vi "IsRequired.vi"(8 "error in":errorcluster, 11 "Control Terminal in":refnum<class "ControlTerminal.lvclass">) -> (0 "error out":errorcluster, 2 "required":bool, 3 "Control Terminal out":refnum<class "ControlTerminal.lvclass">)   [LabVIEW 2014, in "ControlTerminal.lvclass"]
uses:
  ControlTerminal.lvclass
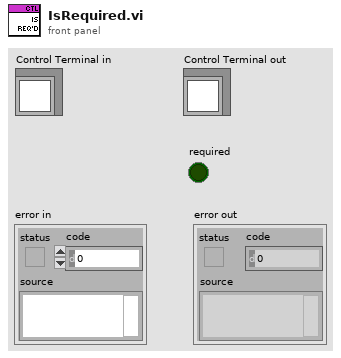
[diagram p1: front panel]
types:
  T1 = enum16{"Invalid Wire Rule", "Required", "Recommended", "Optional", "Dynamic Dispatch"}
  T2 = enum16{"Invalid Wire Rule", "Required", "Recommended", "Optional", "Dynamic Dispatch"}[]
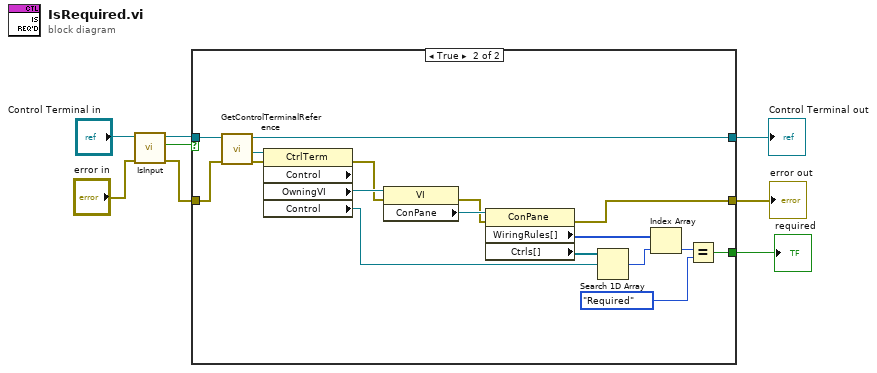
[diagram p0: block diagram]
diagram:
  n1 = call-dynamic "IsInput.vi"("error in"="error in", "ControlTerminal in"="Control Terminal in") -> ("error out"=w2:errorcluster, "input"=w3:bool, "ControlTerminal out"=w4:refnum<class "ControlTerminal.lvclass">)  [unwired: 5 in]
  n2 = case shown="True" w3 {
    tunnel: [w9 w16] -> w8
    tunnel: [_ w17] -> w7
    tunnel: w4 -> [w10 w15]
    tunnel: w2 -> [w9 w14]
    tunnel: [w10 w11] -> w6
    frame False {
    }
    frame True {
      n3 = call "GetControlTerminalReference.vi"("error in"=w14, "ControlTerminal in"=w15) -> ("error out"=w13:errorcluster, "reference"=w12:refnum<vi>, "ControlTerminal out"=w11:refnum<class "ControlTerminal.lvclass">)  [unwired: 7 in]
      n4 = property class="CtrlTerm" props=["Control", "OwningVI", "Control"](reference=w12, error in=w13) -> (error out=w24:errorcluster, "OwningVI"=w27:refnum<vi>, "Control"=w22:refnum<vi>)  [unwired: 2 out]
      n5 = property class="VI"(reference=w27, error in=w24) -> (error out=w25:errorcluster, "ConPane"=w26:refnum<vi>)  [unwired: 1 out]
      n6 = property class="ConPane"(reference=w26, error in=w25) -> (error out=w16:errorcluster, "WiringRules[]"=w21:T2, "Ctrls[]"=w23:refnum<vi>[])  [unwired: 1 out]
      n7 = Search 1D Array(1D array=w23, element=w22) -> (index of element=w20:i32)  [unwired: 1 in]
      n8 = Index Array(array=w21, index=w20) -> (element=w19:T1)
      n9 = Equal?(x=w19, y=T1."Required" ("Wire Rule")) -> (x = y?=w17:bool)
    }
  }
  "error out" <- w8
  "Control Terminal out" <- w6
  "required" <- w7
